vi "Actor Core.vi"(8 "error in":errorcluster, 11 "PredictiveMaintenance in":refnum<class "PredictiveMaintenance.lvclass">) -> (0 "error out":errorcluster, 3 "Actor out":refnum<class "Actor.lvclass">)   [LabVIEW 2019, in "PredictiveMaintenance.lvlib" / "PredictiveMaintenance.lvclass"]
doc: "(<B>Filename</B>: Actor Framework.lvlib:Actor.lvclass:Actor Core.vi)\n\nReceives messages to the actor, reacts to them, and initiates any error handling that may shut the actor down.\n\nDescendant classes may override this VI to append parallel tasks for the actor to complete while it handles messages. Overrides use the Call Parent Method node."
uses:
  PredictiveMaintenance.lvclass
  C:/Program Files (x86)/National Instruments/LabVIEW 2019/vi.lib/ActorFramework/Actor/Actor.lvclass
  <vilib>/ActorFramework/Actor/Actor.lvclass
  typedefs/UI_Control.ctl
  PredictiveMaintenance Messages/Update Msg/Update Msg.lvclass
  C:/Program Files (x86)/National Instruments/LabVIEW 2019/vi.lib/ActorFramework/Message/Message.lvclass
  <vilib>/ActorFramework/Time-Delayed Send Message/Time-Delay Override Options.ctl
  PredictiveMaintenance Messages/Store Msg/Store Msg.lvclass
  PredictiveMaintenance.lvclass/PredictiveMaintenance.ctl
  <vilib>/ActorFramework/Actor/Actor.lvclass/Actor.ctl
  <vilib>/ActorFramework/Message Enqueuer/Message Enqueuer.lvclass/Message Enqueuer.ctl
  PredictiveMaintenance Messages/LimitsVisible Msg/LimitsVisible Msg.lvclass/LimitsVisible Msg.ctl
  <vilib>/ActorFramework/Message Enqueuer/Init from Existing Queue.vi
  <vilib>/ActorFramework/Message Enqueuer/Enqueue.vi
  PredictiveMaintenance Messages/LimitsVisible Msg/LimitsVisible Msg.lvclass
  <vilib>/ActorFramework/Message Priority Queue/Priority Enqueue.vi
  <vilib>/ActorFramework/Message Enqueuer/Message Enqueuer.lvclass
panel:
  in  "show_limits":bool
  out "Events":T1[](array[typedef]) {"err_value" format="%#.0f"; "warn_value" format="%#.0f"; "curr_value" format="%#.0f"; "slider_background" scale=0.0..100.0; "slider" scale=0.0..100.0}
  in  "stop":bool
  out "Trigger":T1[](array[typedef]) {"err_value" format="%#.3f"; "warn_value" format="%#.3f"; "curr_value" format="%#.3f"; "slider_background" scale=0.0..100.0; "slider" scale=0.0..100.0}
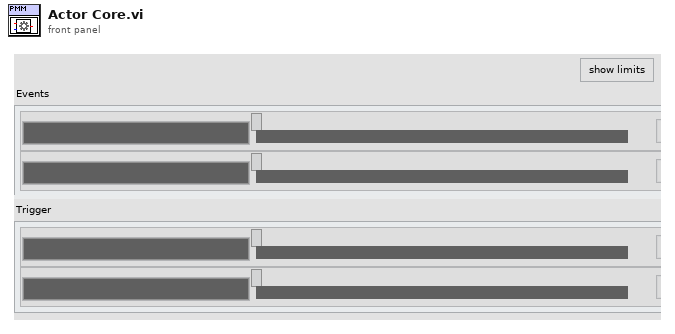
[diagram p1: front panel]
types:
  T1 = typedef "PredictiveMaintenance.lvlib/PredictiveMaintenance.lvclass/UI_Control.ctl" = cluster{"String":string, "slider":dbl, "slider_background":cluster{"Numeric":dbl, "Numeric":dbl, "Numeric":dbl}, "curr_value":dbl, "warn_value":dbl, "err_value":dbl, "colorbox":u32}
  T2 = typedef "Time-Delay Override Options.ctl" = enum16{"Send next copy now", "Skip next scheduled copy", "Send next copy now and stop all further copies", "Stop all further copies"}
  T3 = typedef "LVRectTypeDef.ctl" = cluster{"Left":i16, "Top":i16, "Right":i16, "Bottom":i16}
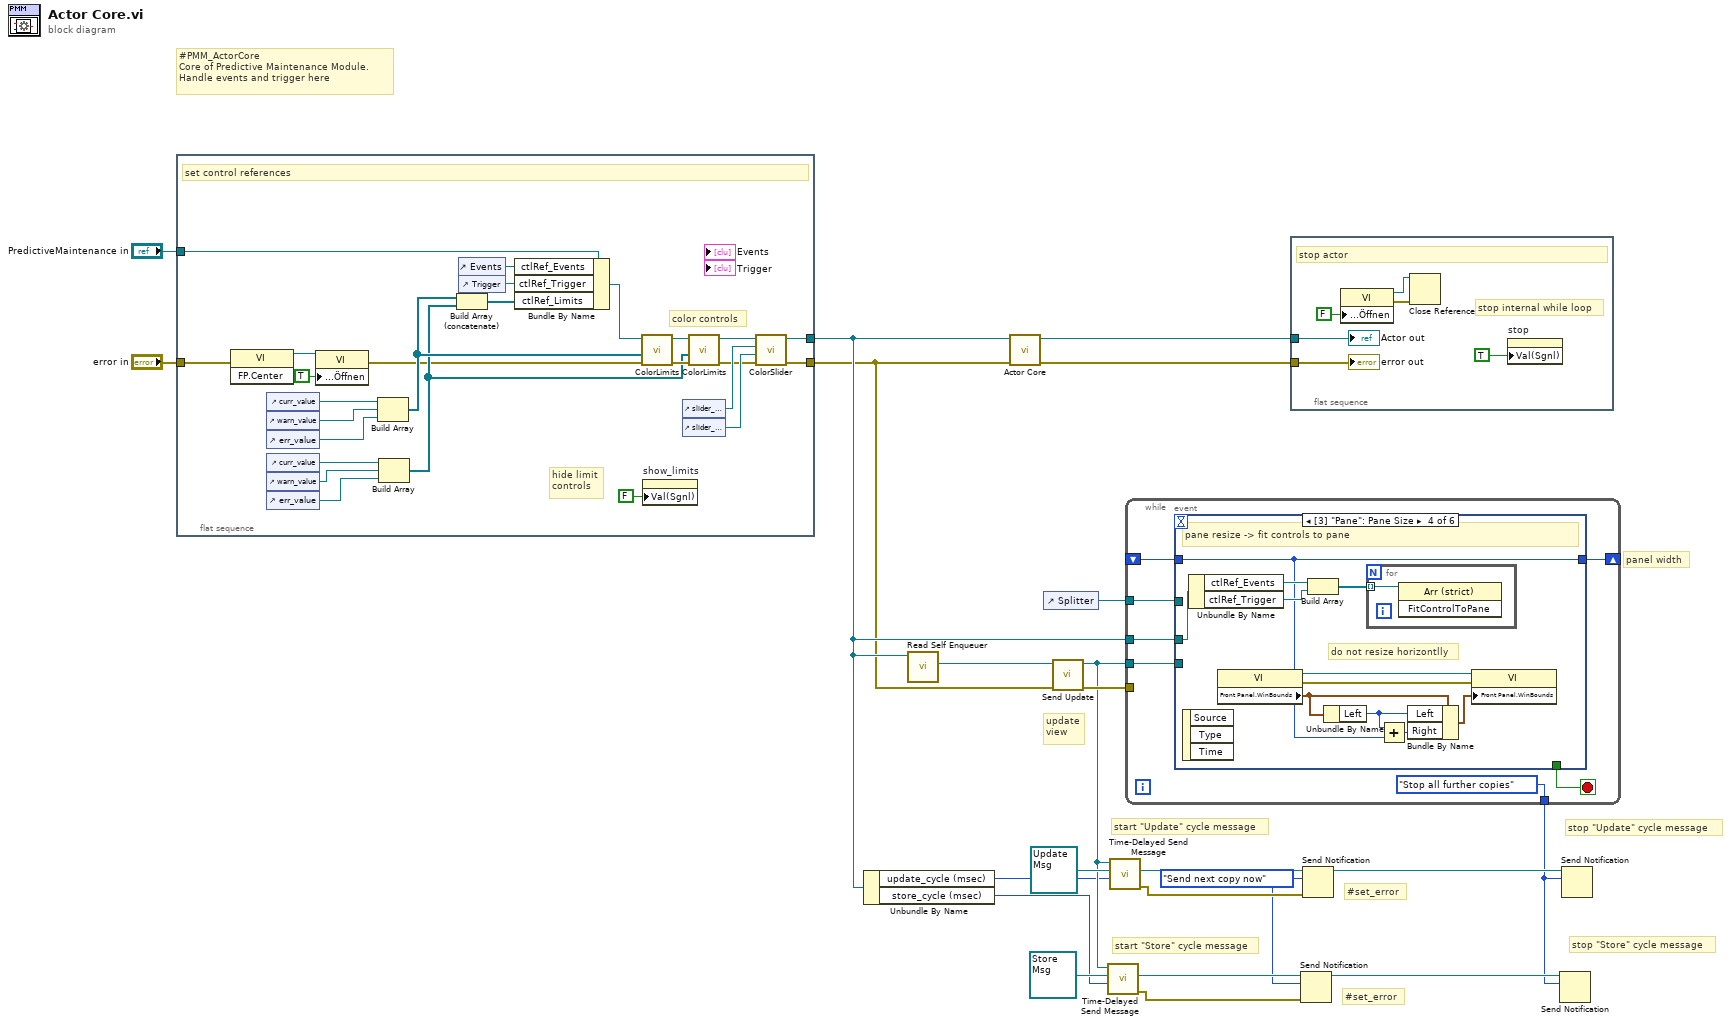
[diagram p0: block diagram]
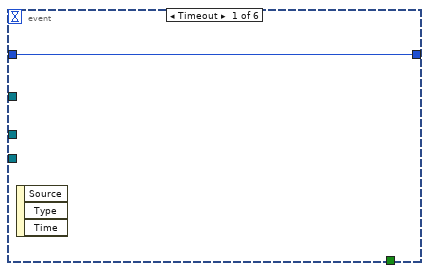
[diagram p2: hidden frame]
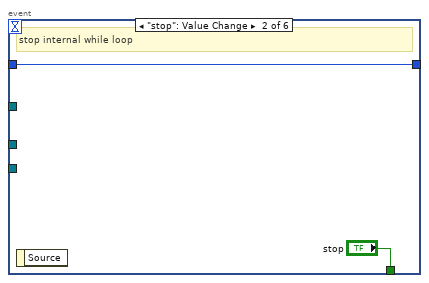
[diagram p3: hidden frame]
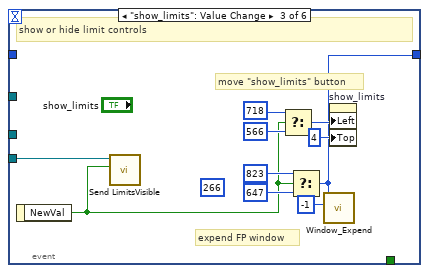
[diagram p4: hidden frame]
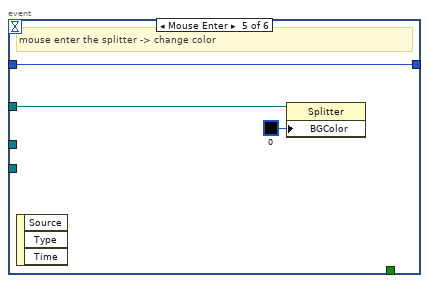
[diagram p5: hidden frame]
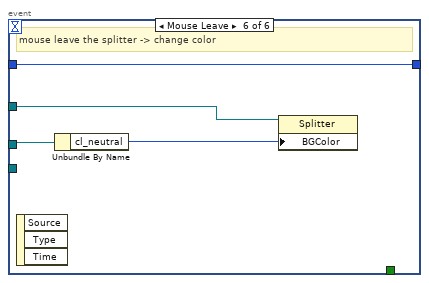
[diagram p6: hidden frame]
diagram:
  w3 = Time-Delay_Override_Options."Send next copy now" ("notification")
  # "panel width"
  # "#PMM_ActorCore\nCore of Predictive Maintenance Module.\nHandle events and trigger here"
  # "update\nview"
  # "stop \"Update\" cycle message"
  # "stop \"Store\" cycle message"
  # "start \"Update\" cycle message"
  # "start \"Store\" cycle message"
  # "#set_error"
  # "#set_error"
  n1 = flat-sequence {
    tunnel: [w36] -> w6
    tunnel: [w28] -> w1
    tunnel: "PredictiveMaintenance in" -> [w39]
    tunnel: "error in" -> [w23]
    frame #0 {
      # "hide limit\ncontrols"
      # "color controls"
      # "set control references"
      n2 = invoke class="VI" method="FP.Center"(error in=w23) -> (reference out=w26:refnum<vi>)  [unwired: 2 in, 2 out]
      n3 = control-ref of="curr_value"() -> (w41:refnum<vi>)
      n4 = control-ref of="warn_value"() -> (w42:refnum<vi>)
      n5 = control-ref of="err_value"() -> (w43:refnum<vi>)
      n6 = control-ref of="curr_value"() -> (w44:refnum<vi>)
      n7 = control-ref of="warn_value"() -> (w45:refnum<vi>)
      n8 = control-ref of="err_value"() -> (w46:refnum<vi>)
      n9 = property class="VI"(reference=w26, "Frontpanel-Fenster:Öffnen"=TRUE ("Front Panel Window:Open")) -> (error out=w24:errorcluster)  [unwired: 1 in, 1 out]
      n10 = Build Array(w41, w42, w43) -> (w30:refnum<vi>[])
      n11 = Build Array(w44, w45, w46) -> (w29:refnum<vi>[])
      n12 = Build Array (concatenate)(w30, w29) -> (w40:refnum<vi>[])
      n13 = control-ref of="Events"() -> (w47:refnum<vi>)
      n14 = control-ref of="Trigger"() -> (w48:refnum<vi>)
      n15 = Bundle By Name(cluster=w39, "ctlRef_Events"=w47, "ctlRef_Trigger"=w48, "ctlRef_Limits"=w40) -> (w32:refnum<class "PredictiveMaintenance.lvclass">)
      n16 = call "ColorLimits.vi"("error in"=w24, "ctlRef_Limits"=w30, "PredictiveMaintenance in"=w32) -> ("error out"=w31:errorcluster, "PredictiveMaintenance OUT"=w33:refnum<class "PredictiveMaintenance.lvclass">)  [unwired: 7 in]
      n17 = property on="show_limits" class="Bool (strict)"("Val(Sgnl)"=FALSE ("Value (Signaling)")) -> ()  [unwired: 2 in, 2 out]
      n18 = control-ref of="slider_background"() -> (w37:refnum<vi>)
      n19 = control-ref of="slider_background"() -> (w38:refnum<vi>)
      n20 = call "ColorLimits.vi"("error in"=w31, "ctlRef_Limits"=w29, "PredictiveMaintenance in"=w33) -> ("error out"=w35:errorcluster, "PredictiveMaintenance OUT"=w34:refnum<class "PredictiveMaintenance.lvclass">)  [unwired: 7 in]
      n21 = call "ColorSlider.vi"("error in (no error)"=w35, "slider_background 2"=w38, "slider_background"=w37, "PredictiveMaintenance in"=w34) -> ("error out"=w28:errorcluster, "PredictiveMaintenance OUT"=w36:refnum<class "PredictiveMaintenance.lvclass">)  [unwired: 6 in]
    }
  }
  n22 = Unbundle By Name(w6) -> ("update_cycle (msec)"=w5:i32, "store_cycle (msec)"=w4:i32)
  n23 = call <vilib>:"Read Self Enqueuer.vi"("Actor"=w6) -> ("Self Enqueuer"=w2:refnum<class "Message Enqueuer.lvclass">)  [unwired: 10 in]
  n24 = call-parent "Actor Core.vi"("error in"=w1, "Actor in"=w6) -> ("error out"=w22:errorcluster, "Actor out"=w21:refnum<class "Actor.lvclass">)  [unwired: 8 in]
  n25 = control-ref of="Splitter"() -> (w20:refnum<vi>)
  n26 = call "Send Update.vi"("error in (no error)"=w1, "Message Enqueuer"=w2) -> ("error out"=w19:errorcluster, "Message Enqueuer out"=w8:refnum<class "Message Enqueuer.lvclass">)  [unwired: 8 in]
  n27 = call <vilib>:"Time-Delayed Send Message.vi"("Milliseconds To Wait"=w4, "Message"=refnum<class "Store Msg.lvclass"> refnum ("PredictiveMaintenance.lvlib:Store Msg.lvclass"), "Message Enqueuer"=w8) -> ("error out"=w12:errorcluster, "Delivery Notifier"=w10:refnum<notifier>)  [unwired: 7 in]
  n28 = call <vilib>:"Time-Delayed Send Message.vi"("Milliseconds To Wait"=w5, "Message"=refnum<class "Update Msg.lvclass"> refnum ("Message Type"), "Message Enqueuer"=w8) -> ("error out"=w13:errorcluster, "Delivery Notifier"=w15:refnum<notifier>)  [unwired: 7 in]
  n29 = while {
    tunnel: w8 -> [w54]
    tunnel: w6 -> [w53]
    tunnel: w20 -> [w52]
    tunnel: w19 -> [_]
    tunnel: [Time-Delay_Override_Options."Stop all further copies" ("notification")] -> w7
    shift-right: [w50] -> _
    shift-left: _ -> [w49]
    stop <- w55 stop-if-true
    n30 = event shown="[3] \"Pane\": Pane Size" {
      selector: _ -> [_ _ _ _ _ _]
      dyn-events: _ -> [_ _ _ _ _ _]
      timeout: _ -> [_ _ _ _ _ _]
      tunnel: [_ "stop" _ _ _ _] -> w55
      tunnel: w54 -> [_ _ w68 _ _ _]
      tunnel: w53 -> [_ _ _ w79 _ w86]
      tunnel: w52 -> [_ _ _ _ w83 w87]
      tunnel: [w56 w57 w59 w70 w81 w84] -> w50
      tunnel: w49 -> [w56 w57 _ w70 w81 w84]
      event Timeout {
        n31 = event-data() -> ()  [unwired: 1 in, 3 out]
      }
      event "stop": Value Change {
        # "stop internal while loop"
        n32 = event-data() -> ()  [unwired: 1 in, 1 out]
      }
      event "show_limits": Value Change {
        (unwired) i16 266 ("height")
        # "move \"show_limits\" button"
        # "expend FP window"
        # "show or hide limit controls"
        n33 = event-data() -> ("NewVal"=w60:bool)  [unwired: 1 in]
        n34 = call "Send LimitsVisible.vi"("visible?"=w60, "Message Enqueuer"=w68) -> ()  [unwired: 8 in, 2 out]
        n35 = Select(t=718 ("Position:Top"), s=w60, f=566) -> (s? t:f=w66:i32)
        n36 = Select(t=i16 823 ("width"), s=w60, f=i16 647) -> (s? t:f=w59:i16)
        n37 = call "Window_Expend.vi"("height"=i16 -1, "width"=w59) -> ()  [unwired: 9 in, 1 out]
        n38 = property on="show_limits" class="Bool (strict)"("Left"=w66, "Top"=4 ("Position:Top")) -> ()  [unwired: 2 in, 2 out]
      }
      event Pane Size {
        # "do not resize horizontlly"
        # "pane resize -> fit controls to pane"
        n39 = event-data() -> ()  [unwired: 1 in, 3 out]
        n40 = Unbundle By Name(w79) -> ("ctlRef_Events"=w78:refnum<vi>, "ctlRef_Trigger"=w76:refnum<vi>)
        n41 = property class="VI"() -> (reference out=w71:refnum<vi>, error out=w73:errorcluster, "Front Panel.WinBounds"=w74:T3)  [unwired: 2 in]
        n42 = Build Array(w78, w76) -> (w77:refnum<vi>[])
        n43 = Unbundle By Name(w74) -> ("Left"=w69:i16)
        n44 = for {
          tunnel: w77 -> [w80] mode=indexing
          n45 = invoke class="Arr (strict)" method="FitControlToPane"(reference=w80) -> ()  [unwired: 2 in, 3 out]
        }
        n46 = Add(x=w69, y=w70) -> (x+y=w75:i16)
        n47 = Bundle By Name(cluster=w74, "Left"=w69, "Right"=w75) -> (w72:T3)
        n48 = property class="VI"(reference=w71, error in=w73, "Front Panel.WinBounds"=w72) -> ()  [unwired: 2 out]
      }
      event Mouse Enter {
        # "mouse enter the splitter -> change color"
        n49 = event-data() -> ()  [unwired: 1 in, 3 out]
        n50 = property class="Splitter"(reference=w83, "BGColor"=u32 0 ("Colors:BG Color")) -> ()  [unwired: 1 in, 2 out]
      }
      event Mouse Leave {
        # "mouse leave the splitter -> change color"
        n51 = event-data() -> ()  [unwired: 1 in, 3 out]
        n52 = Unbundle By Name(w86) -> ("cl_neutral"=w85:u32)
        n53 = property class="Splitter"(reference=w87, "BGColor"=w85) -> ()  [unwired: 1 in, 2 out]
      }
    }
  }
  n54 = flat-sequence {
    tunnel: w22 -> [w93]
    tunnel: w21 -> [w92]
    frame #0 {
      # "stop internal while loop"
      # "stop actor"
      n55 = property class="VI"("Frontpanel-Fenster:Öffnen"=FALSE ("Front Panel Window:Open")) -> (reference out=w89:refnum<vi>, error out=w90:errorcluster)  [unwired: 2 in]
      n56 = Close Reference(reference=w89, error in (no error)=w90) -> ()  [unwired: 1 out]
      n57 = property on="stop" class="Bool (strict)"("Val(Sgnl)"=TRUE ("Value (Signaling)")) -> ()  [unwired: 2 in, 2 out]
      "error out" <- w93
      "Actor out" <- w92
    }
  }
  n58 = Send Notification(notification=w3, notifier=w10, error in (no error)=w12) -> (notifier out=w11:refnum<notifier>)  [unwired: 1 out]
  n59 = Send Notification(notification=w3, notifier=w15, error in (no error)=w13) -> (notifier out=w14:refnum<notifier>)  [unwired: 1 out]
  n60 = Send Notification(notification=w7, notifier=w11) -> ()  [unwired: 1 in, 2 out]
  n61 = Send Notification(notification=w7, notifier=w14) -> ()  [unwired: 1 in, 2 out]
